vi "Read Qsp.vi"(8 "error in (no error)":errorcluster, 11 "VC Data in":refnum<class "VC Data.lvclass">) -> (0 "error out":errorcluster, 2 "Qsp":sgl, 3 "VC Data out":refnum<class "VC Data.lvclass">)   [LabVIEW 2014, in "VC Data.lvclass"]
uses:
  VC Data.lvclass
  VC Data.lvclass/VC Data.ctl
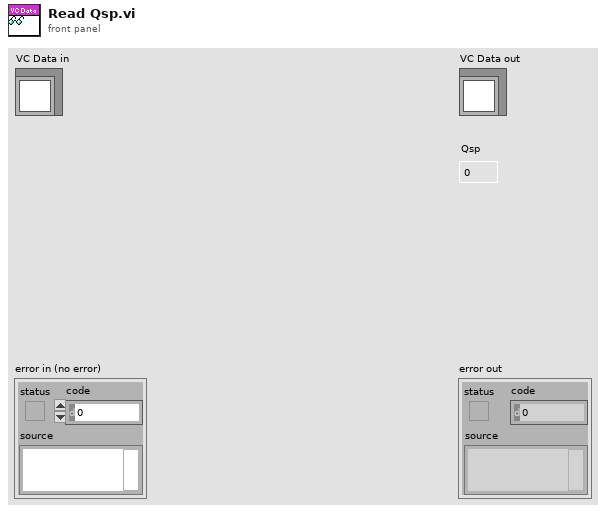
[diagram p1: front panel]
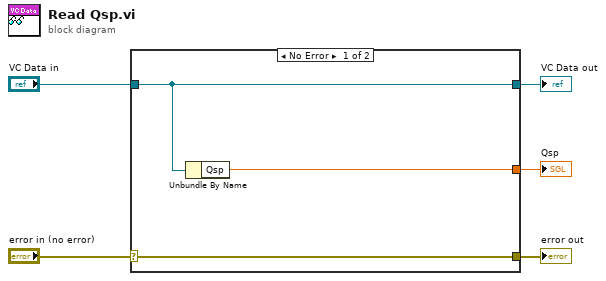
[diagram p0: block diagram]
diagram:
  n1 = case shown="No Error" "error in (no error)" {
    selector: "error in (no error)" -> [w8 w9]
    tunnel: [w8 w9] -> w4
    tunnel: [w7 w10] -> w2
    tunnel: "VC Data in" -> [w7 w10]
    tunnel: [w6 _] -> w1
    frame No Error {
      n2 = Unbundle By Name(w7) -> ("Qsp"=w6:sgl)
    }
    frame Error {
    }
  }
  "error out" <- w4
  "VC Data out" <- w2
  "Qsp" <- w1
